vi "DIMPowerSupply.ConvertMonitor.vi"(0 "i ref in":refnum<vi>, 2 "moduleValue":dbl, 5 "error in (no error)":errorcluster) -> (14 "i ref out":refnum<vi>, 16 "actual PS voltage [V]":dbl format="%.2f", 19 "error out":errorcluster)   [LabVIEW 2014, in "DIMPowerSupply.lvlib"]
doc: "Converts the number output of the module (typically a 16bit unsigned integer) to the actual value [V] of the power supply."
uses:
  DIMPowerSupply.lvlib
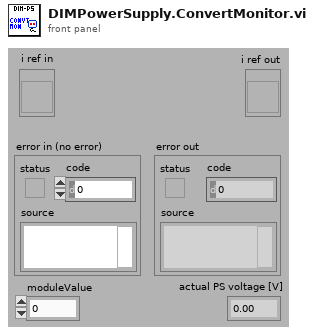
[diagram p1: front panel]
types:
  T1 = typedef "DIMPowerSupply.lvlib/DIMPowerSupply.ranges type.ctl" = cluster{"deviceMin":dbl, "deviceMax":dbl, "numberMin":u16, "numberMax":u16, "U16?":bool, "factor":dbl}
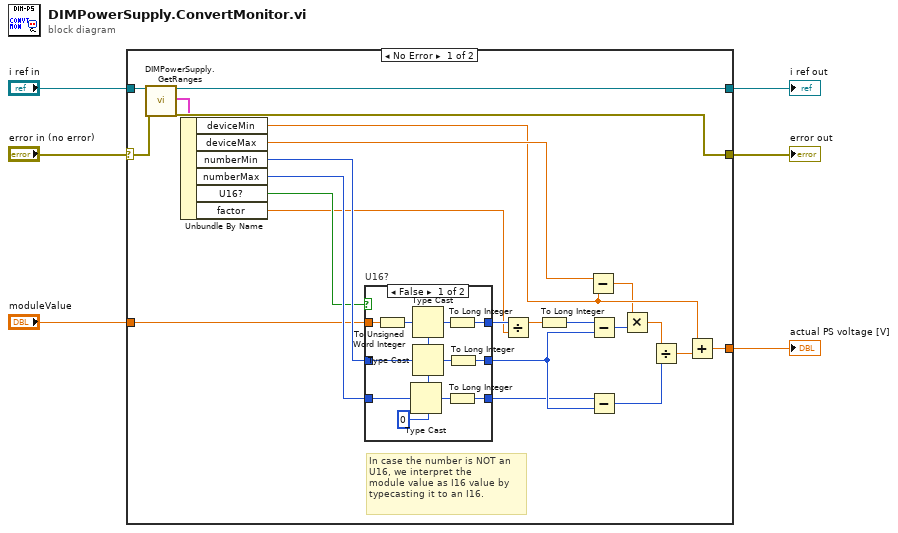
[diagram p0: block diagram]
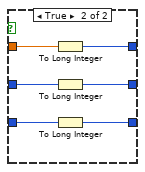
[diagram p2: hidden frame]
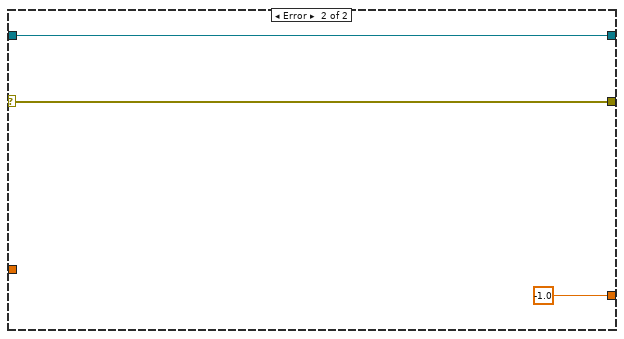
[diagram p3: hidden frame]
diagram:
  n1 = case shown="No Error" "error in (no error)" {
    selector: "error in (no error)" -> [w20 w48]
    tunnel: "i ref in" -> [w29 w49]
    tunnel: [w28 w49] -> w5
    tunnel: [w27 w48] -> w4
    tunnel: "moduleValue" -> [w11 _]
    tunnel: [w21 -1.0] -> w2
    frame No Error {
      # "In case the number is NOT an\nU16, we interpret the\nmodule value as I16 value by\ntypecasting it to an I16."
      n2 = call "DIMPowerSupply.GetRanges.vi"("i ref in"=w29, "error in (no error)"=w20) -> ("i ref out"=w28:refnum<vi>, "MonitorRanges"=w26:T1, "error out"=w27:errorcluster)  [unwired: 14 in, 1 out]
      n3 = Unbundle By Name(w26) -> ("deviceMin"=w24:dbl, "deviceMax"=w25:dbl, "numberMin"=w23:u16, "numberMax"=w22:u16, "U16?"=w12:bool, "factor"=w9:dbl)
      n4 = case "U16?" shown="False" w12 {
        tunnel: w23 -> [w40 w46]
        tunnel: w22 -> [w39 w44]
        tunnel: [w36 w45] -> w14
        tunnel: [w35 w43] -> w13
        tunnel: [w31 w41] -> w10
        tunnel: w11 -> [w34 w42]
        frame False {
          w32 = i16 0
          n5 = To Unsigned Word Integer(number=w34) -> (unsigned 16bit integer=w33:u16)
          n6 = Type Cast(type=w32, x=w39) -> (*(type *) &x=w37:i16)
          n7 = Type Cast(type=w32, x=w33) -> (*(type *) &x=w30:i16)
          n8 = Type Cast(type=w32, x=w40) -> (*(type *) &x=w38:i16)
          n9 = To Long Integer(number=w30) -> (32bit integer=w31:i32)
          n10 = To Long Integer(number=w37) -> (32bit integer=w35:i32)
          n11 = To Long Integer(number=w38) -> (32bit integer=w36:i32)
        }
        frame True {
          n12 = To Long Integer(number=w42) -> (32bit integer=w41:i32)
          n13 = To Long Integer(number=w46) -> (32bit integer=w45:i32)
          n14 = To Long Integer(number=w44) -> (32bit integer=w43:i32)
        }
      }
      n15 = Divide(x=w10, y=w9) -> (x/y=w8:dbl)
      n16 = To Long Integer(number=w8) -> (32bit integer=w7:i32)
      n17 = Subtract(x=w25, y=w24) -> (x-y=w19:dbl)
      n18 = Subtract(x=w7, y=w14) -> (x-y=w18:i32)
      n19 = Subtract(x=w13, y=w14) -> (x-y=w16:i32)
      n20 = Multiply(x=w19, y=w18) -> (x*y=w17:dbl)
      n21 = Divide(x=w17, y=w16) -> (x/y=w15:dbl)
      n22 = Add(x=w24, y=w15) -> (x+y=w21:dbl)
    }
    frame Error {
    }
  }
  "error out" <- w4
  "i ref out" <- w5
  "actual PS voltage [V]" <- w2
